vi "Destroy User Event - ExitEventLoop.vi"(8 "error in (no error)":errorcluster, 10 "user event ExitEventLoop":refnum<user-event>) -> (0 "error out":errorcluster)   [LabVIEW 2017, in "UserEvent-ExitEventLoop.lvlib"]
doc: "Destroy the user event, even if there is an incoming error.\n\nBolder Software LLC"
uses:
  UserEvent-ExitEventLoop.lvlib
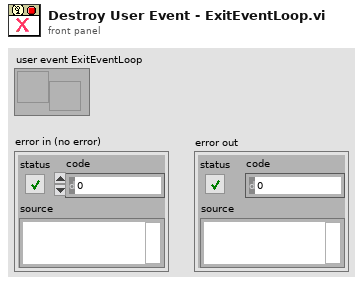
[diagram p1: front panel]
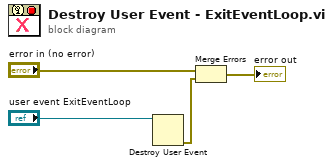
[diagram p0: block diagram]
diagram:
  n1 = Destroy User Event(user event="user event ExitEventLoop") -> (error out=w4:errorcluster)  [unwired: 1 in]
  n2 = Merge Errors("error in (no error)", w4) -> (→"error out":errorcluster)
